vi "Front Panel DataSocket - Reader.vi"() -> ()   [LabVIEW 2023]
doc: "Uses DataSocket to subscribe to data. The waveform graph on the front panel subscribes to the DataSocket Server on the local computer. When the VI runs, the indicator connects to the DataSocket Server and acquires data from it.\n\nTo set up the DataSocket connection of the waveform graph, right-click the waveform graph and select Properties and go to the Data Binding tab."
panel:
  in  "Stop":bool
  out "Data Read":dbl[](graph)
  # "Overview: Demonstrates the use of DataSocket front panel binding to read data from the DataSocket server.\nRequirements: Windows\nInstructions:\n1. Ensure Front Panel DataSocket - Writer.vi is already running.\n2. Run the VI.\n3. Click Stop to stop the VI."
  # "Right-click the graph and choose Properties, then select the Data Binding tab, to configure the graph to read its data from the DataSocket server. This graph is configured to read data from the following URL:\n\ndstp://localhost/fpwave\n\nNote that the connection status LED in the upper-right corner of the graph will turn green when the VI runs and a DataSocket connection is established."
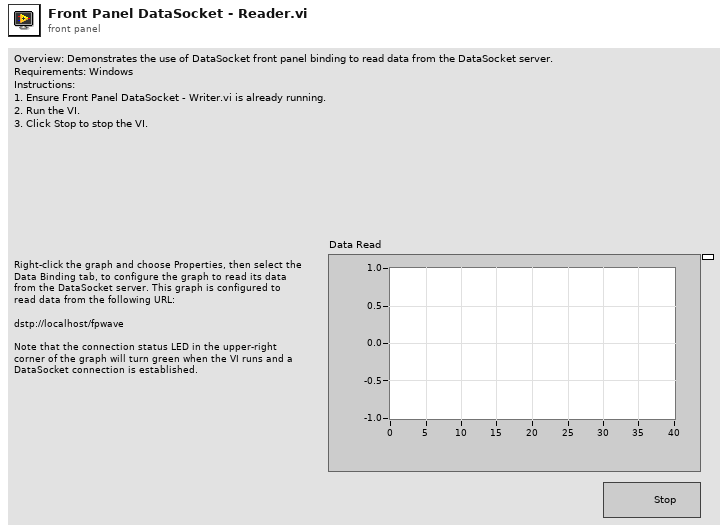
[diagram p1: front panel]
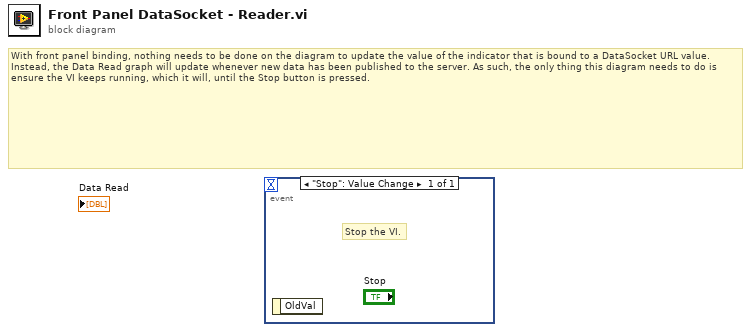
[diagram p0: block diagram]
diagram:
  # "With front panel binding, nothing needs to be done on the diagram to update the value of the indicator that is bound to a DataSocket URL value. Instead, the Data Read graph will update whenever new data has been published to the server. As such, the only thing this diagram needs to do is ensure the VI keeps running, which it will, until the Stop button is pressed."
  n1 = event shown="[0] \"Stop\": Value Change" {
    selector: _ -> [_]
    dyn-events: _ -> [_]
    timeout: _ -> [_]
    event "Stop": Value Change {
      # "Stop the VI."
      n2 = event-data() -> ()  [unwired: 1 in, 1 out]
    }
  }
